vi "compress_local_messages.vi"(8 "error in (no error)":errorcluster, 10 "ok message":string="Z1:00000001000000000200000000030000000004000000000500000000060000000007000000000800000000092345", 11 "header":string="XX00.XX00.XX00.XX00.XX00") -> (0 "error out":errorcluster, 3 "message":string)   [LabVIEW 2019, in "Messages.lvlib"]
uses:
  Messages.lvlib
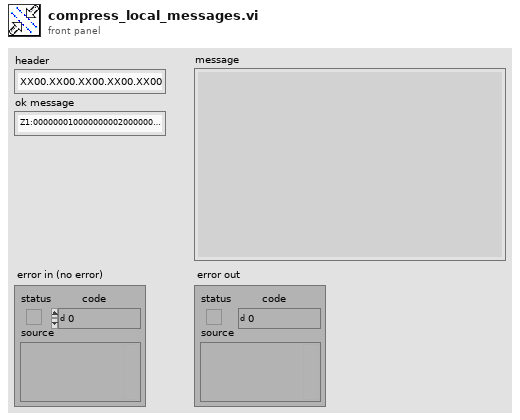
[diagram p1: front panel]
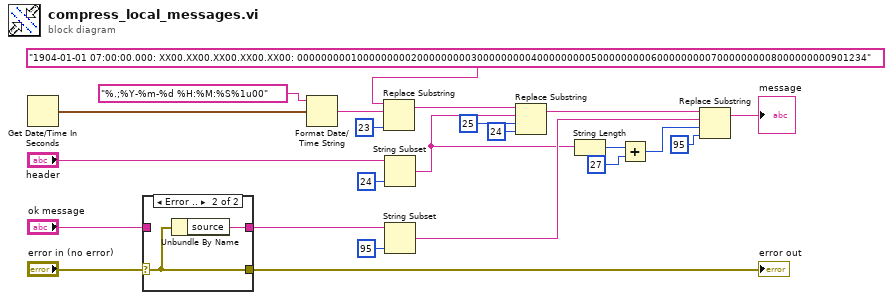
[diagram p0: block diagram]
diagram:
  n1 = Get Date/Time In Seconds() -> (seconds since 1Jan1904=w1:timestamp)
  n2 = case shown="Error .." "error in (no error)" {
    selector: "error in (no error)" -> [w24 w26]
    tunnel: [w25 w27] -> w9
    tunnel: "ok message" -> [w25 _]
    tunnel: [w24 w26] -> w8
    frame No Error {
    }
    frame Error {
      n3 = Unbundle By Name(w26) -> ("source"=w27:string)
    }
  }
  "error out" <- w8
  n4 = Format Date/Time String(time format string (%c)="%.;%Y-%m-%d %H:%M:%S%1u00", seconds (now)=w1) -> (date/time string=w2:string)  [unwired: 1 in]
  n5 = Replace Substring(2:23 ("x+y"), 4:w2, 5:"1904-01-01 07:00:00.000: XX00.XX00.XX00.XX00.XX00: 00000000010000000002000000000300000000040000000005000000000600000000070000000008000000000901234" ("object 3")) -> (1:w5:string)  [unwired: 1 in, 1 out]
  n6 = String Subset(string="header", length (rest)=24 ("length (rest)")) -> (substring=w15:string)  [unwired: 1 in]
  n7 = String Subset(string=w9, length (rest)=95 ("length (rest)")) -> (substring=w22:string)  [unwired: 1 in]
  n8 = Replace Substring(2:24 ("x+y"), 3:25 ("offset (0)"), 4:w15, 5:w5) -> (1:w19:string)  [unwired: 1 out]
  n9 = String Length(string=w15) -> (length=w14:i32)
  n10 = Add(x=w14, y=27 ("value")) -> (x+y=w18:i32)
  n11 = Replace Substring(2:95 ("x+y"), 3:w18, 4:w22, 5:w19) -> (1:→"message":string)  [unwired: 1 out]
